vi "System5.vi"() -> ()   [LabVIEW 2015]
uses:
  Control 1.ctl
  <vilib>/DAQmx/read.llb/DAQmx Read (Analog 1D Wfm NChan NSamp).vi
  <vilib>/DAQmx/write.llb/DAQmx Write (Digital 1D Bool NChan 1Samp 1Line).vi
  <vilib>/Analysis/baseanly.llb/Mean (DBL).vi
  <vilib>/DAQmx/write.llb/DAQmx Write (Analog DBL 1Chan 1Samp).vi
  <vilib>/DAQmx/miscellaneous.llb/DAQmx Fill In Error Info.vi
  <vilib>/addons/control/pid/NI_PID_autopid.lvlib
  <vilib>/Analysis/NI_AALBase.lvlib
panel:
  in  "Open/Close (Green)":bool
  in  "Open/Close (Blue)":bool
  in  "Stop program":bool
  in  "On/Off":bool
  in  "Manual Control 2":bool
  in  "Voltage setting 2":dbl format="%#_13g"
  out "Voltage Reading(pressure) 2":dbl format="%#_13g"
  out "Pressure 2":dbl format="%#.3g"
  out "Pressure Chart 2":dbl(graph)
  in  "autotuning parameters 2":T1={"controller type"=1, "relay cycles"=3, "relay amplitude"=1.0, "control specification"=2, "PV noise level"=0.1} {"PV noise level" format="%.2f"; "control specification" items=["normal", "fast", "slow"]; "relay amplitude" format="%.2f"; "controller type" items=["PID", "PI", "P"]}
  in  "PID gains 2":T2={"proportional gain (Kc)"=1.0, "integral time (Ti, min)"=0.01, "derivative time (Td, min)"=0.0} {"derivative time (Td, min)" format="%.3f"; "integral time (Ti, min)" format="%.3f"; "proportional gain (Kc)" format="%.3f"}
  out "PID gains out 2":T2={"proportional gain (Kc)"=1.0, "integral time (Ti, min)"=0.01, "derivative time (Td, min)"=0.0} {"derivative time (Td, min)" format="%.3f"; "integral time (Ti, min)" format="%.3f"; "proportional gain (Kc)" format="%.3f"}
  in  "autotune? (F) 2":bool
  in  "reinitialize? (F) 2":bool
  in  "setpoint in Bar 2":dbl format="%#.5f"
  out "Control Value 2":dbl
  in  "Voltage setting":dbl format="%#_13g"
  in  "Manual Control":bool
  out "Control Value":dbl
  in  "setpoint in Bar":dbl format="%#.5f"
  in  "reinitialize? (F)":bool
  in  "autotune? (F)":bool
  out "PID gains out":T2={"proportional gain (Kc)"=1.0, "integral time (Ti, min)"=0.01, "derivative time (Td, min)"=0.0} {"derivative time (Td, min)" format="%.3f"; "integral time (Ti, min)" format="%.3f"; "proportional gain (Kc)" format="%.3f"}
  in  "PID gains":T2={"proportional gain (Kc)"=1.0, "integral time (Ti, min)"=0.01, "derivative time (Td, min)"=0.0} {"derivative time (Td, min)" format="%.3f"; "integral time (Ti, min)" format="%.3f"; "proportional gain (Kc)" format="%.3f"}
  in  "autotuning parameters":T1={"controller type"=1, "relay cycles"=3, "relay amplitude"=1.0, "control specification"=2, "PV noise level"=0.1} {"PV noise level" format="%.2f"; "control specification" items=["normal", "fast", "slow"]; "relay amplitude" format="%.2f"; "controller type" items=["PID", "PI", "P"]}
  out "Pressure Chart":dbl(graph)
  out "Pressure":dbl format="%#.3g"
  out "Voltage Reading(pressure)":dbl format="%#_13g"
  # "Pressure Vessel 2"
  # "Pressure Vessel 1"
  # "Readings"
  # "Controls"
  # "Readings"
  # "Controls"
  # "PID Settings"
  # "51.12139\n\n0.044676"
  # "Valves"
  # "Pump 3"
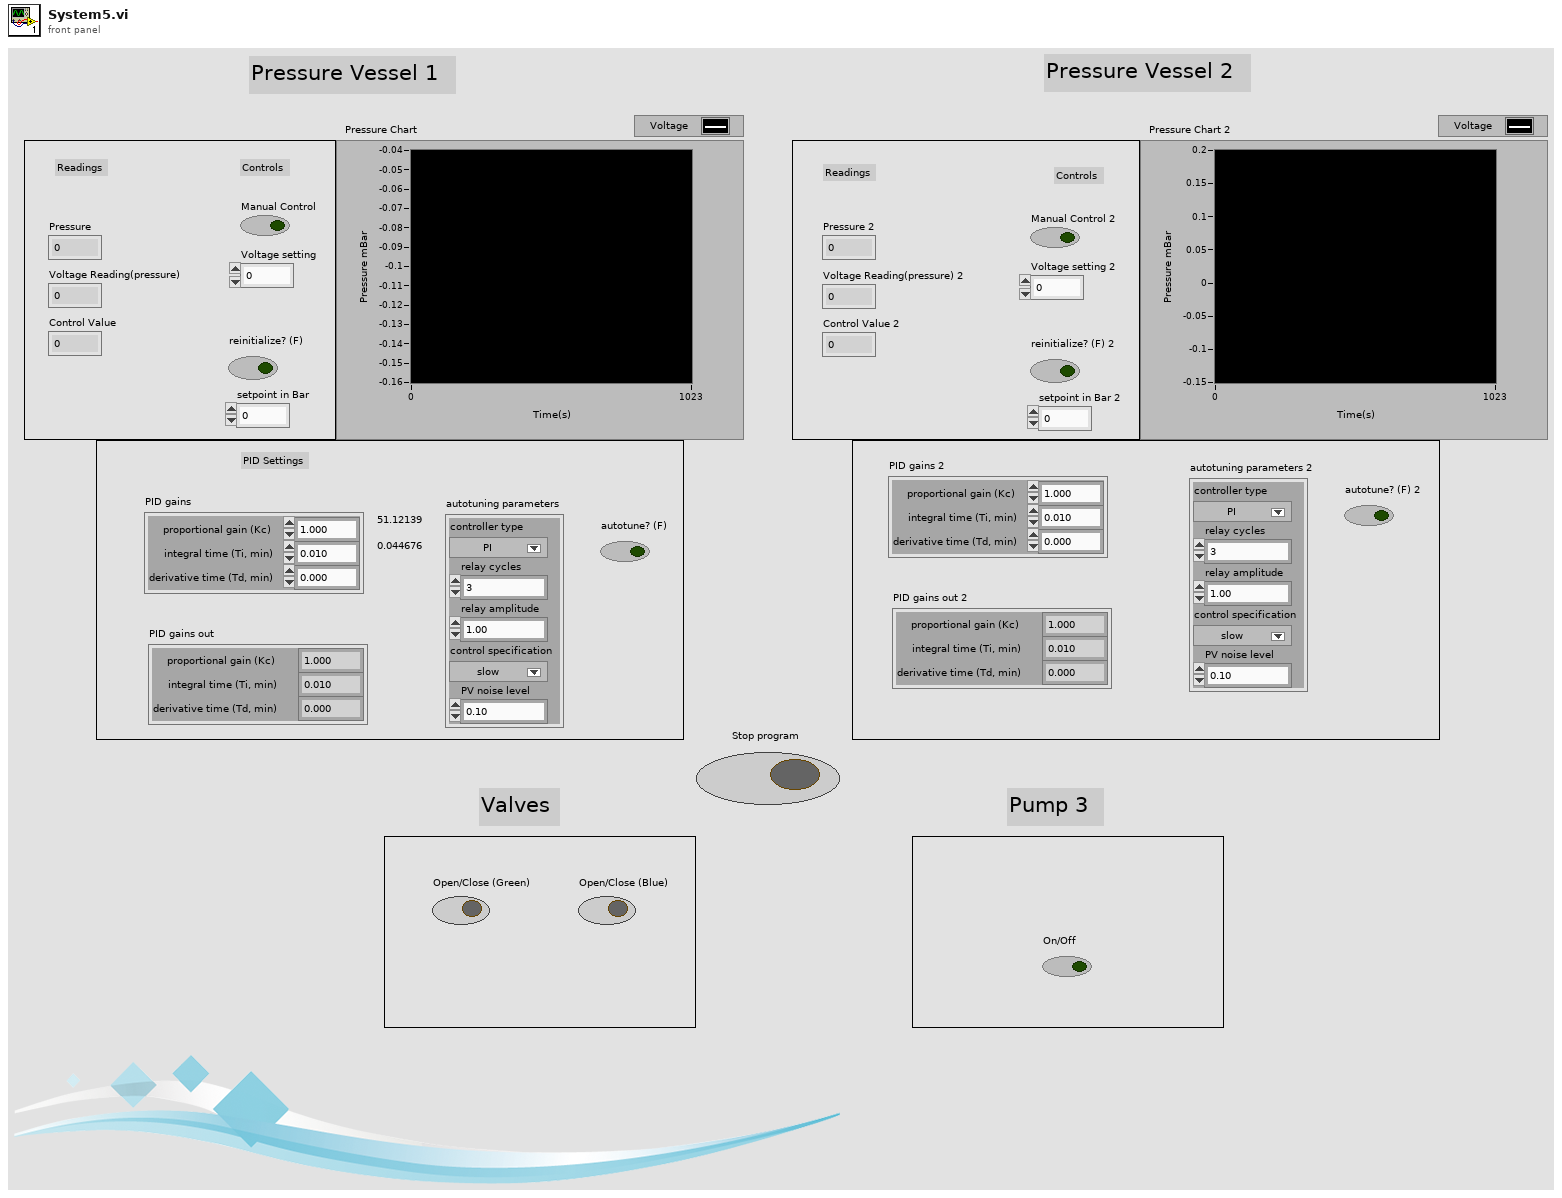
[diagram p1: front panel]
types:
  T1 = cluster{"controller type":u16, "relay cycles":i32, "relay amplitude":dbl, "control specification":u16, "PV noise level":dbl}
  T2 = cluster{"proportional gain (Kc)":dbl, "integral time (Ti, min)":dbl, "derivative time (Td, min)":dbl}
  T3 = typedef "Control 1.ctl" = refnum<k21>
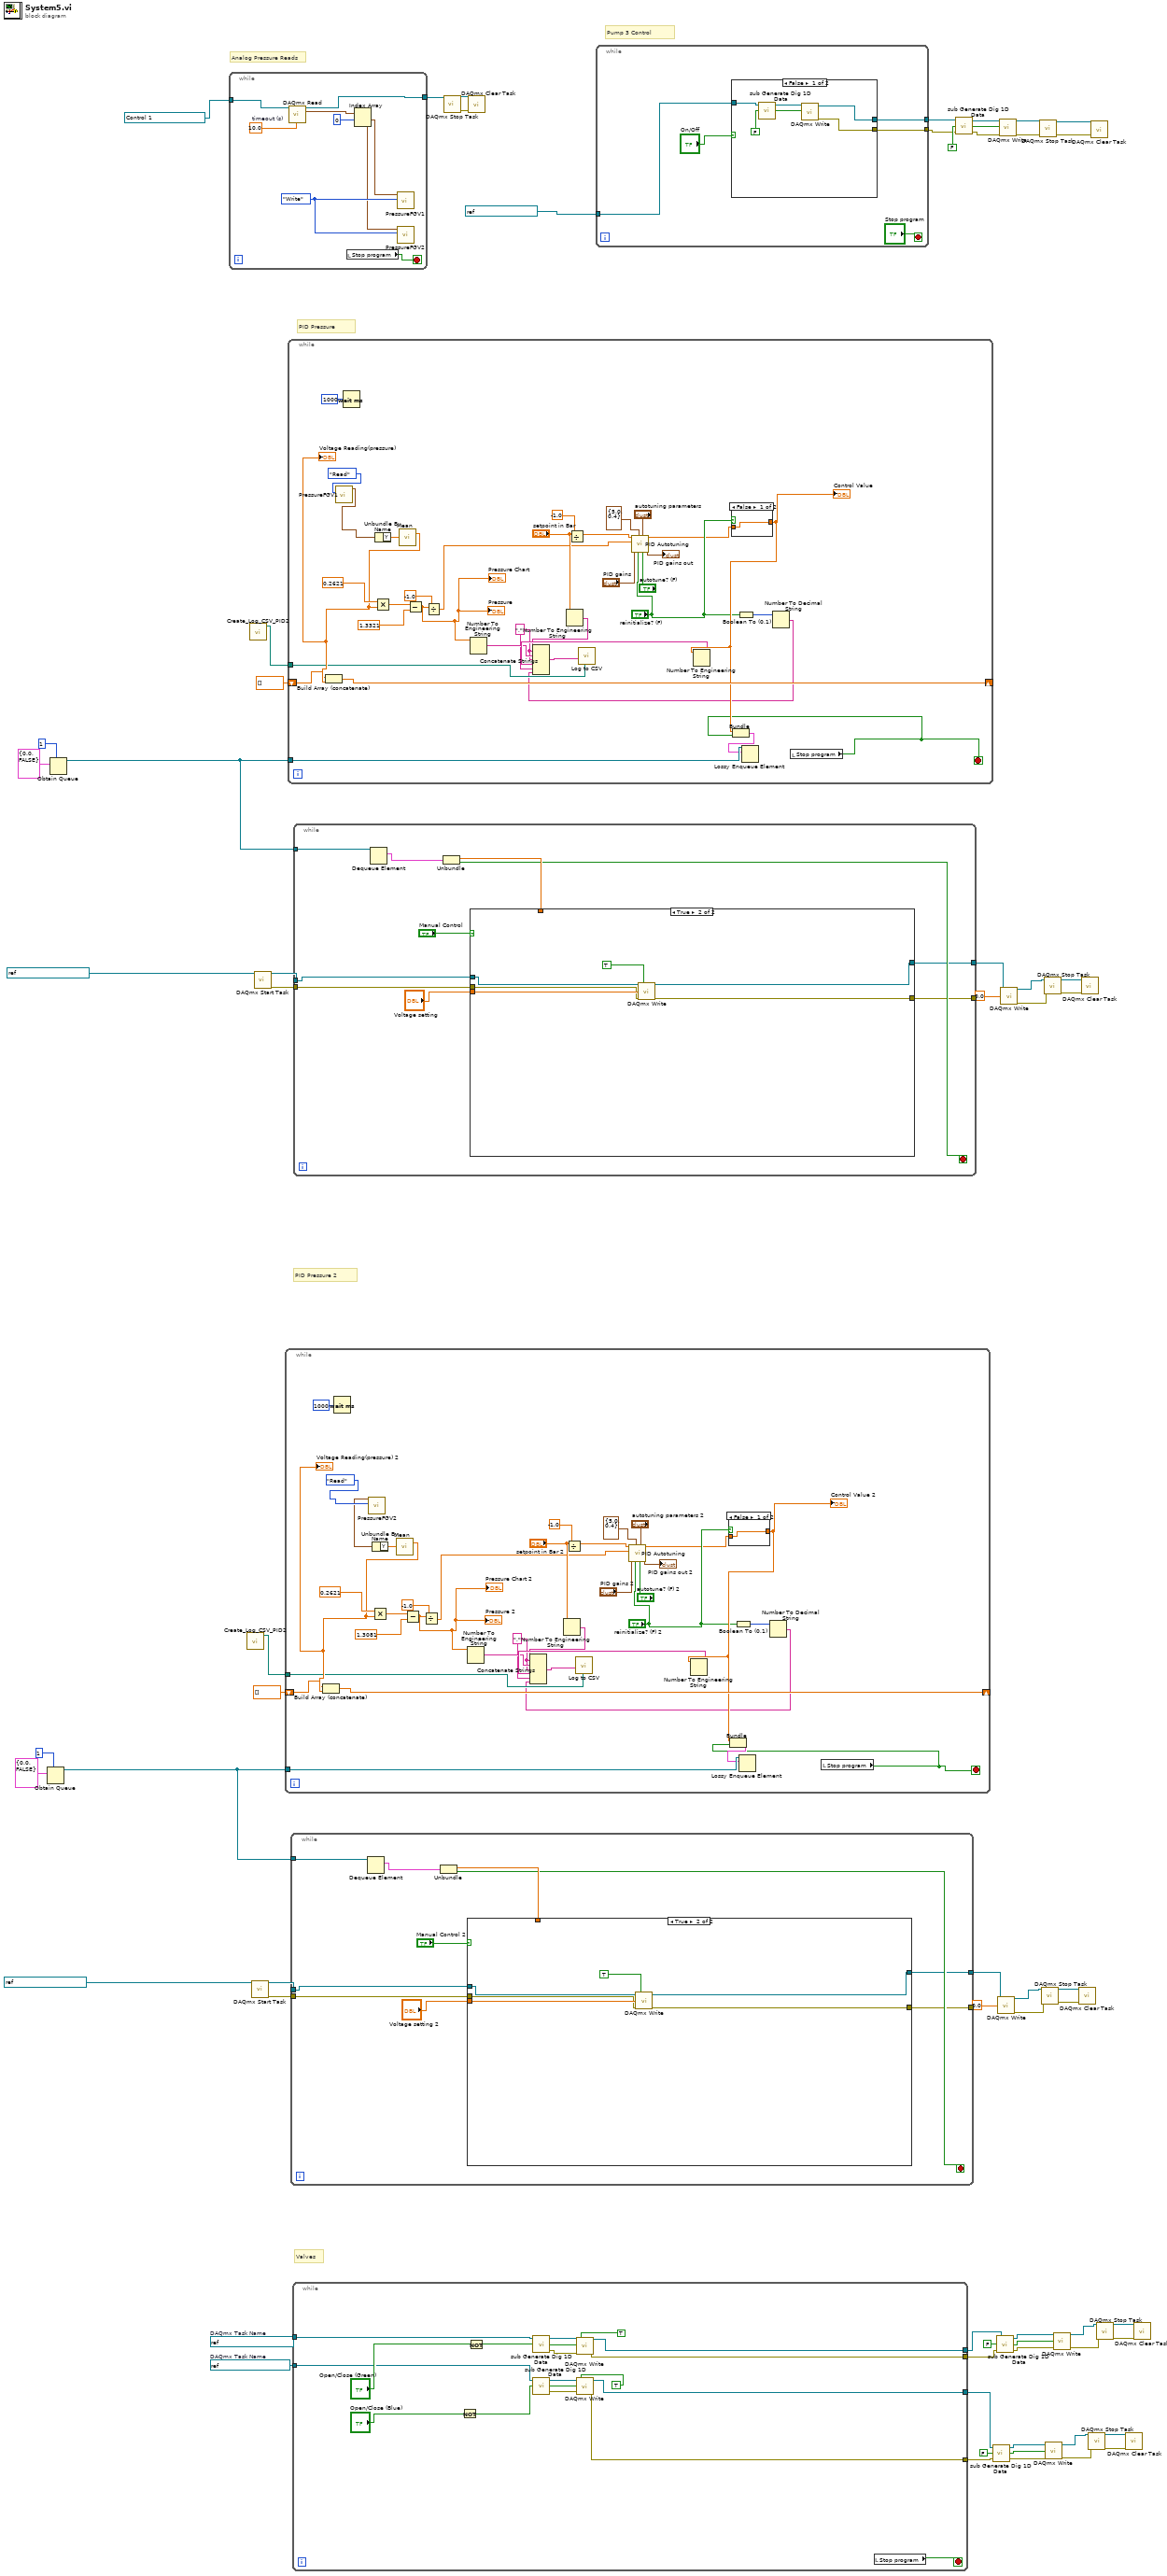
[diagram p0: block diagram]
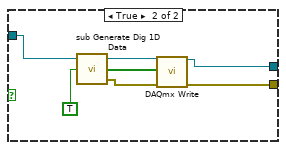
[diagram p2: hidden frame]
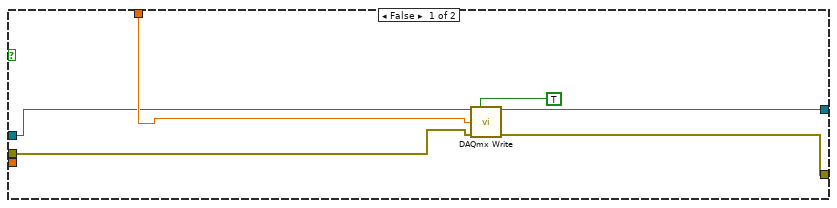
[diagram p3: hidden frame]
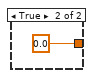
[diagram p4: hidden frame]
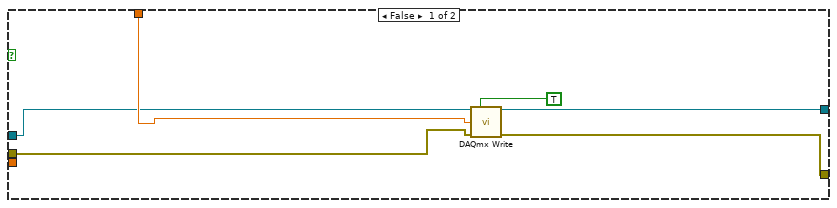
[diagram p5: hidden frame]
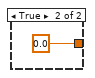
[diagram p6: hidden frame]
diagram:
  w25 = refnum<k21> "NewDigitalSystemBlue"  # DAQmx Task Name
  w26 = refnum<k21> "NewDigitalSystemGreen"  # DAQmx Task Name
  # "Analog Pressure Reads"
  # "Valves"
  # "Pump 3 Control"
  # "PID Pressure"
  # "PID Pressure 2"
  n1 = Obtain Queue(max queue size (-1, unlimited)=1, element data type=cluster{dbl, bool} {0.0, FALSE}) -> (queue out=w50:refnum<queue>)  [unwired: 3 in, 2 out]
  n2 = Obtain Queue(max queue size (-1, unlimited)=1, element data type=cluster{dbl, bool} {0.0, FALSE}) -> (queue out=w64:refnum<queue>)  [unwired: 3 in, 2 out]
  n3 = while {
    tunnel: T3 "New AnalogSystemAI0" -> [w72]
    tunnel: [w71] -> w1
    stop <- w74 stop-if-true
    w68 = enum16{"Write", "Read"}."Write" ("Command")
    w73 = 10.0  # timeout (s)
    n4 = call-poly <vilib>:"DAQmx Read.vi"("task/channels in"=w72, "timeout"=w73) -> ("task out"=w71:refnum<k21>, "data"=w69:waveform(dbl)[])  [unwired: 11 in, 1 out]
    n5 = local read "Stop program"() -> (w74:bool)
    n6 = Index Array(array=w69, index #1=0 ("index")) -> (element #1=w67:waveform(dbl), element #2=w66:waveform(dbl))  [unwired: 1 in]
    n7 = call "PressureFGV1.vi"("Command"=w68, "element"=w67) -> ()  [unwired: 9 in, 1 out]
    n8 = call "PressureFGV2.vi"("Command"=w68, "element"=w66) -> ()  [unwired: 9 in, 1 out]
  }
  n9 = call "Create_Log_CSV_PID2.vi"() -> ("path"=w46:path)  [unwired: 11 in]
  n10 = call "Create_Log_CSV_PID2.vi"() -> ("path"=w60:path)  [unwired: 11 in]
  n11 = call <vilib>:"DAQmx Start Task.vi"("task/channels in"=refnum<k21> "NewAnalogSystemAO1") -> ("task out"=w45:refnum<k21>, "error out"=w44:errorcluster)  [unwired: 13 in]
  n12 = call <vilib>:"DAQmx Start Task.vi"("task/channels in"=refnum<k21> "NewAnalogSystemAO0") -> ("task out"=w59:refnum<k21>, "error out"=w58:errorcluster)  [unwired: 13 in]
  n13 = while {
    tunnel: w50 -> [w101]
    shift-right: [w98] -> _
    shift-left: dbl[] [] -> [w99]
    tunnel: w46 -> [w92]
    stop <- w79 stop-if-true
    w87 = ","
    n14 = Wait (ms)(milliseconds to wait=u32 1000) -> ()  [unwired: 1 out]
    n15 = call "PressureFGV2.vi"("Command"=enum16{"Write", "Read"}."Read") -> ("element 2"=w75:waveform(dbl))  [unwired: 10 in]
    n16 = Unbundle By Name(w75) -> ("Y"=w77:dbl[])
    n17 = call-poly <vilib>:"Mean.vi"("X"=w77) -> ("mean"=w100:dbl)  [unwired: 1 out]
    "Voltage Reading(pressure) 2" <- w100
    n18 = Build Array (concatenate)(w99, w100) -> (w98:dbl[])
    n19 = Multiply(x=0.2621, y=w100) -> (x*y=w108:dbl)
    n20 = Subtract(x=w108, y=1.3081) -> (x-y=w96:dbl)
    "Pressure 2" <- w96
    "Pressure Chart 2" <- w96
    n21 = Divide(x=w96, y=-1.0) -> (x/y=w84:dbl)
    n22 = Number To Engineering String(4:w96) -> (0:w91:string)  [unwired: 3 in]
    n23 = Number To Engineering String(4:"setpoint in Bar 2") -> (0:w90:string)  [unwired: 3 in]
    n24 = Divide(x="setpoint in Bar 2", y=-1.0) -> (x/y=w83:dbl)
    n25 = call <vilib>:"PID Autotuning.vi"("autotune? (F)"="autotune? (F) 2", "autotuning parameters"="autotuning parameters 2", "reinitialize? (F)"="reinitialize? (F) 2", "output range"=cluster{"output high":dbl, "output low":dbl} {"output high"=5.0, "output low"=0.4}, "PID gains"="PID gains 2", "process variable"=w84, "setpoint"=w83) -> ("PID gains out"=→"PID gains out 2":T2, "output"=w81:dbl)  [unwired: 1 in, 2 out]
    n26 = case shown="False" "reinitialize? (F) 2" {
      tunnel: [w110 0.0] -> w95
      tunnel: w81 -> [w110 _]
      frame False {
      }
      frame True {
      }
    }
    "Control Value 2" <- w95
    n27 = Number To Engineering String(4:w95) -> (0:w94:string)  [unwired: 3 in]
    n28 = Boolean To (0,1)(Boolean="reinitialize? (F) 2") -> (0, 1=w88:i16)
    n29 = Number To Decimal String(number=w88) -> (decimal integer string=w86:string)  [unwired: 1 in]
    n30 = Concatenate Strings(w90, w87, w91, w87, w94, w87, w86) -> (w93:string)
    n31 = call "Log to CSV.vi"("Data Str"=w93, "Path"=w92) -> ()  [unwired: 5 in, 1 out]
    n32 = local read "Stop program"() -> (w79:bool)
    n33 = Bundle("output"=w95, "Stop program"=w79) -> (w80:cluster{"output":dbl, "Stop program":bool})  [unwired: 1 in]
    n34 = Lossy Enqueue Element(queue=w101, element=w80) -> ()  [unwired: 1 in, 4 out]
  }
  n35 = while {
    tunnel: w64 -> [w138]
    shift-right: [w133] -> _
    shift-left: dbl[] [] -> [w134]
    tunnel: w60 -> [w127]
    stop <- w115 stop-if-true
    w122 = ","
    n36 = call "PressureFGV1.vi"("Command"=enum16{"Write", "Read"}."Read") -> ("element 2"=w112:waveform(dbl))  [unwired: 10 in]
    n37 = Wait (ms)(milliseconds to wait=u32 1000) -> ()  [unwired: 1 out]
    n38 = Unbundle By Name(w112) -> ("Y"=w136:dbl[])
    n39 = call-poly <vilib>:"Mean.vi"("X"=w136) -> ("mean"=w135:dbl)  [unwired: 1 out]
    "Voltage Reading(pressure)" <- w135
    n40 = Build Array (concatenate)(w134, w135) -> (w133:dbl[])
    n41 = Multiply(x=0.2621, y=w135) -> (x*y=w145:dbl)
    n42 = Subtract(x=w145, y=1.3321) -> (x-y=w131:dbl)
    "Pressure" <- w131
    "Pressure Chart" <- w131
    n43 = Divide(x=w131, y=-1.0) -> (x/y=w119:dbl)
    n44 = Number To Engineering String(4:w131) -> (0:w126:string)  [unwired: 3 in]
    n45 = Number To Engineering String(4:"setpoint in Bar") -> (0:w125:string)  [unwired: 3 in]
    n46 = Divide(x="setpoint in Bar", y=-1.0) -> (x/y=w118:dbl)
    n47 = call <vilib>:"PID Autotuning.vi"("autotune? (F)"="autotune? (F)", "autotuning parameters"="autotuning parameters", "reinitialize? (F)"="reinitialize? (F)", "output range"=cluster{"output high":dbl, "output low":dbl} {"output high"=5.0, "output low"=0.4}, "PID gains"="PID gains", "process variable"=w119, "setpoint"=w118) -> ("PID gains out"=→"PID gains out":T2, "output"=w116:dbl)  [unwired: 1 in, 2 out]
    n48 = case shown="False" "reinitialize? (F)" {
      tunnel: [w147 0.0] -> w130
      tunnel: w116 -> [w147 _]
      frame False {
      }
      frame True {
      }
    }
    "Control Value" <- w130
    n49 = Number To Engineering String(4:w130) -> (0:w129:string)  [unwired: 3 in]
    n50 = Boolean To (0,1)(Boolean="reinitialize? (F)") -> (0, 1=w123:i16)
    n51 = Number To Decimal String(number=w123) -> (decimal integer string=w121:string)  [unwired: 1 in]
    n52 = Concatenate Strings(w125, w122, w126, w122, w129, w122, w121) -> (w128:string)
    n53 = call "Log to CSV.vi"("Data Str"=w128, "Path"=w127) -> ()  [unwired: 5 in, 1 out]
    n54 = local read "Stop program"() -> (w115:bool)
    n55 = Bundle("output"=w130, "Stop program"=w115) -> (w137:cluster{"output":dbl, "Stop program":bool})  [unwired: 1 in]
    n56 = Lossy Enqueue Element(queue=w138, element=w137) -> ()  [unwired: 1 in, 4 out]
  }
  n57 = while {
    tunnel: w50 -> [w158]
    tunnel: w45 -> [w156]
    tunnel: [w151] -> w42
    tunnel: w44 -> [w150]
    tunnel: [w149] -> _
    stop <- w152 stop-if-true
    n58 = Dequeue Element(queue=w158) -> (element=w155:cluster{dbl, bool})  [unwired: 2 in, 3 out]
    n59 = Unbundle(w155) -> (w154:dbl, w152:bool)
    n60 = case shown="True" "Manual Control 2" {
      tunnel: w156 -> [w162 w169]
      tunnel: w154 -> [w163 _]
      tunnel: "Voltage setting 2" -> [_ w168]
      tunnel: [w161 w167] -> w151
      tunnel: w150 -> [w160 w166]
      tunnel: [w159 w165] -> w149
      frame False {
        n61 = call-poly <vilib>:"DAQmx Write.vi"("task/channels in"=w162, "auto start"=TRUE, "data"=w163, "error in"=w160) -> ("task out"=w161:refnum<k21>, "error out"=w159:errorcluster)  [unwired: 9 in, 1 out]
      }
      frame True {
        n62 = call-poly <vilib>:"DAQmx Write.vi"("task/channels in"=w169, "auto start"=TRUE, "data"=w168, "error in"=w166) -> ("task out"=w167:refnum<k21>, "error out"=w165:errorcluster)  [unwired: 9 in, 1 out]
      }
    }
  }
  n63 = while {
    tunnel: w26 -> [w179]
    tunnel: w25 -> [w178]
    tunnel: [w177] -> w15
    tunnel: [w176] -> w11
    tunnel: [w173] -> w8
    tunnel: [w172] -> w6
    stop <- w171 stop-if-true
    n64 = Not(x="Open/Close (Blue)") -> (.not. x?=w189:bool)
    n65 = Not(x="Open/Close (Green)") -> (.not. x?=w188:bool)
    n66 = call <vilib>:"sub Generate Dig 1D Data.vi"("initial value"=w188, "task in"=w179) -> ("error out"=w175:errorcluster, "Data"=w186:bool[], "task out"=w183:refnum<k21>)  [unwired: 1 in]
    n67 = call <vilib>:"sub Generate Dig 1D Data.vi"("initial value"=w189, "task in"=w178) -> ("error out"=w174:errorcluster, "Data"=w185:bool[], "task out"=w184:refnum<k21>)  [unwired: 1 in]
    n68 = call-poly <vilib>:"DAQmx Write.vi"("task/channels in"=w183, "auto start"=TRUE, "data"=w186, "error in"=w175) -> ("task out"=w177:refnum<k21>, "error out"=w173:errorcluster)  [unwired: 9 in, 1 out]
    n69 = call-poly <vilib>:"DAQmx Write.vi"("task/channels in"=w184, "auto start"=TRUE, "data"=w185, "error in"=w174) -> ("task out"=w176:refnum<k21>, "error out"=w172:errorcluster)  [unwired: 9 in, 1 out]
    n70 = local read "Stop program"() -> (w171:bool)
  }
  n71 = while {
    tunnel: w64 -> [w199]
    tunnel: w59 -> [w197]
    tunnel: [w192] -> w56
    tunnel: w58 -> [w191]
    tunnel: [w190] -> _
    stop <- w193 stop-if-true
    n72 = Dequeue Element(queue=w199) -> (element=w196:cluster{dbl, bool})  [unwired: 2 in, 3 out]
    n73 = Unbundle(w196) -> (w195:dbl, w193:bool)
    n74 = case shown="True" "Manual Control" {
      tunnel: w197 -> [w203 w210]
      tunnel: w195 -> [w204 _]
      tunnel: "Voltage setting" -> [_ w209]
      tunnel: [w202 w208] -> w192
      tunnel: w191 -> [w201 w207]
      tunnel: [w200 w206] -> w190
      frame False {
        n75 = call-poly <vilib>:"DAQmx Write.vi"("task/channels in"=w203, "auto start"=TRUE, "data"=w204, "error in"=w201) -> ("task out"=w202:refnum<k21>, "error out"=w200:errorcluster)  [unwired: 9 in, 1 out]
      }
      frame True {
        n76 = call-poly <vilib>:"DAQmx Write.vi"("task/channels in"=w210, "auto start"=TRUE, "data"=w209, "error in"=w207) -> ("task out"=w208:refnum<k21>, "error out"=w206:errorcluster)  [unwired: 9 in, 1 out]
      }
    }
  }
  n77 = call <vilib>:"DAQmx Stop Task.vi"("task/channels in"=w1) -> ("task out"=w3:refnum<k21>, "error out"=w2:errorcluster)  [unwired: 13 in]
  n78 = call <vilib>:"DAQmx Clear Task.vi"("task in"=w3, "error in"=w2) -> ()  [unwired: 13 in, 1 out]
  n79 = while {
    tunnel: refnum<k21> "NewDigSystemP0L2" -> [w215]
    tunnel: [w214] -> w30
    tunnel: [w213] -> w29
    stop <- "Stop program" stop-if-true
    n80 = case shown="False" "On/Off" {
      tunnel: w215 -> [w222 w226]
      tunnel: [w218 w225] -> w214
      tunnel: [w217 w223] -> w213
      frame False {
        n81 = call <vilib>:"sub Generate Dig 1D Data.vi"("initial value"=FALSE, "task in"=w222) -> ("Data"=w220:bool[], "task out"=w221:refnum<k21>)  [unwired: 1 in, 1 out]
        n82 = call-poly <vilib>:"DAQmx Write.vi"("task/channels in"=w221, "data"=w220) -> ("task out"=w218:refnum<k21>, "error out"=w217:errorcluster)  [unwired: 11 in, 1 out]
      }
      frame True {
        n83 = call <vilib>:"sub Generate Dig 1D Data.vi"("initial value"=TRUE, "task in"=w226) -> ("error out"=w224:errorcluster, "Data"=w228:bool[], "task out"=w227:refnum<k21>)  [unwired: 1 in]
        n84 = call-poly <vilib>:"DAQmx Write.vi"("task/channels in"=w227, "data"=w228, "error in"=w224) -> ("task out"=w225:refnum<k21>, "error out"=w223:errorcluster)  [unwired: 10 in, 1 out]
      }
    }
  }
  n85 = call <vilib>:"sub Generate Dig 1D Data.vi"("error in"=w29, "initial value"=FALSE, "task in"=w30) -> ("error out"=w34:errorcluster, "Data"=w32:bool[], "task out"=w33:refnum<k21>)
  n86 = call <vilib>:"sub Generate Dig 1D Data.vi"("error in"=w6, "initial value"=FALSE, "task in"=w11) -> ("error out"=w5:errorcluster, "Data"=w10:bool[], "task out"=w12:refnum<k21>)
  n87 = call <vilib>:"sub Generate Dig 1D Data.vi"("error in"=w8, "initial value"=FALSE, "task in"=w15) -> ("error out"=w7:errorcluster, "Data"=w9:bool[], "task out"=w16:refnum<k21>)
  n88 = call-poly <vilib>:"DAQmx Write.vi"("task/channels in"=w42, "data"=0.0) -> ("task out"=w41:refnum<k21>, "error out"=w40:errorcluster)  [unwired: 11 in, 1 out]
  n89 = call-poly <vilib>:"DAQmx Write.vi"("task/channels in"=w33, "data"=w32, "error in"=w34) -> ("task out"=w28:refnum<k21>, "error out"=w27:errorcluster)  [unwired: 10 in, 1 out]
  n90 = call-poly <vilib>:"DAQmx Write.vi"("task/channels in"=w56, "data"=0.0) -> ("task out"=w55:refnum<k21>, "error out"=w54:errorcluster)  [unwired: 11 in, 1 out]
  n91 = call <vilib>:"DAQmx Stop Task.vi"("task/channels in"=w28, "error in"=w27) -> ("task out"=w36:refnum<k21>, "error out"=w35:errorcluster)  [unwired: 12 in]
  n92 = call <vilib>:"DAQmx Stop Task.vi"("task/channels in"=w41, "error in"=w40) -> ("task out"=w43:refnum<k21>, "error out"=w39:errorcluster)  [unwired: 12 in]
  n93 = call <vilib>:"DAQmx Stop Task.vi"("task/channels in"=w55, "error in"=w54) -> ("task out"=w57:refnum<k21>, "error out"=w53:errorcluster)  [unwired: 12 in]
  n94 = call-poly <vilib>:"DAQmx Write.vi"("task/channels in"=w12, "data"=w10, "error in"=w5) -> ("task out"=w19:refnum<k21>, "error out"=w18:errorcluster)  [unwired: 10 in, 1 out]
  n95 = call-poly <vilib>:"DAQmx Write.vi"("task/channels in"=w16, "data"=w9, "error in"=w7) -> ("task out"=w22:refnum<k21>, "error out"=w23:errorcluster)  [unwired: 10 in, 1 out]
  n96 = call <vilib>:"DAQmx Clear Task.vi"("task in"=w43, "error in"=w39) -> ()  [unwired: 13 in, 1 out]
  n97 = call <vilib>:"DAQmx Clear Task.vi"("task in"=w57, "error in"=w53) -> ()  [unwired: 13 in, 1 out]
  n98 = call <vilib>:"DAQmx Stop Task.vi"("task/channels in"=w19, "error in"=w18) -> ("task out"=w20:refnum<k21>, "error out"=w17:errorcluster)  [unwired: 12 in]
  n99 = call <vilib>:"DAQmx Clear Task.vi"("task in"=w36, "error in"=w35) -> ()  [unwired: 13 in, 1 out]
  n100 = call <vilib>:"DAQmx Stop Task.vi"("task/channels in"=w22, "error in"=w23) -> ("task out"=w21:refnum<k21>, "error out"=w24:errorcluster)  [unwired: 12 in]
  n101 = call <vilib>:"DAQmx Clear Task.vi"("task in"=w20, "error in"=w17) -> ()  [unwired: 13 in, 1 out]
  n102 = call <vilib>:"DAQmx Clear Task.vi"("task in"=w21, "error in"=w24) -> ()  [unwired: 13 in, 1 out]
